vi "Reset State.vi"(8 "error in (no error)":errorcluster, 11 "LoggingControl in":refnum<class "LoggingControl.lvclass">) -> (0 "error out":errorcluster, 3 "LoggingControl out":refnum<class "LoggingControl.lvclass">)   [LabVIEW 2020, in "VolatusGUIElements.lvlib" / "LoggingControl.lvclass"]
uses:
  LoggingControl.lvclass
  LoggingControl.lvclass/LoggingControl.ctl
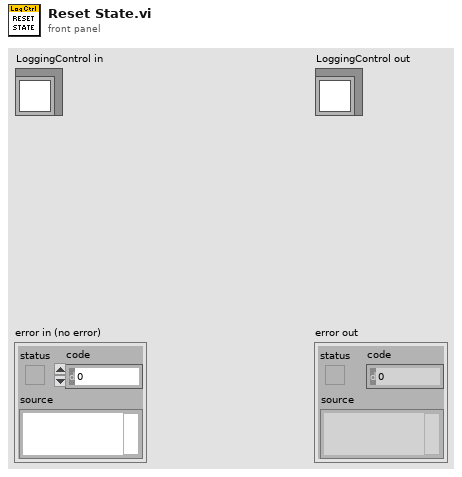
[diagram p1: front panel]
types:
  T1 = typedef "VolatusGUIElements.lvlib/LoggingControl.lvclass/Log State.ctl" = cluster{"Series":string, "Timestamp":string, "Requested":bool}
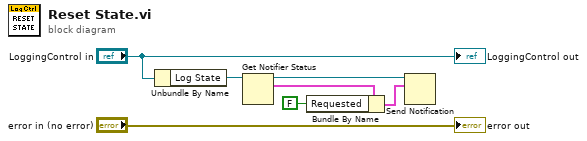
[diagram p0: block diagram]
diagram:
  n1 = Unbundle By Name("LoggingControl in") -> ("Log State"=w5:refnum<notifier>)
  n2 = Get Notifier Status(notifier=w5) -> (notifier out=w2:refnum<notifier>, current notification=w4:T1)  [unwired: 1 in, 3 out]
  n3 = Bundle By Name(cluster=w4, "Requested"=FALSE) -> (w1:T1)
  n4 = Send Notification(notification=w1, notifier=w2) -> ()  [unwired: 1 in, 2 out]
  "error out" <- "error in (no error)"
  "LoggingControl out" <- "LoggingControl in"
